vi "piezoUSBWriteWaveform.vi"(1 "positions (um)":dbl[](array[numeric])) -> ()   [LabVIEW 2017]
uses:
  globalDevices.vi
  Piezo/lvlib/Madlib.lvlib
panel:
  out "function return 2":i32
  out "Waveform Graph":dbl[](graph)
  out "function return":i32
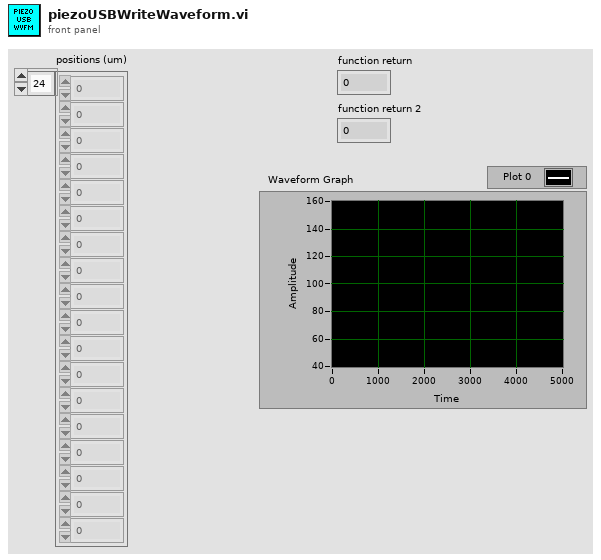
[diagram p1: front panel]
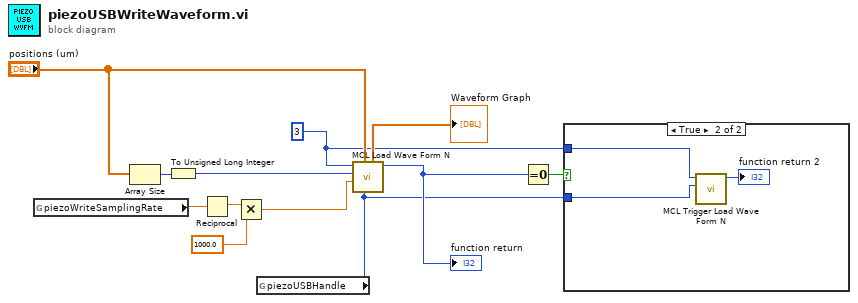
[diagram p0: block diagram]
diagram:
  w2 = u32 3 ("axis")
  n1 = global read "globalDevices.vi" "piezoWriteSamplingRate"() -> (w9:dbl)
  n2 = Array Size(array="positions (um)") -> (size(s)=w11:i32)
  n3 = To Unsigned Long Integer(number=w11) -> (unsigned 32bit integer=w10:u32)
  n4 = Reciprocal(x=w9) -> (1/x=w8:dbl)
  n5 = Multiply(x=w8, y=1000.0) -> (x*y=w6:dbl)
  n6 = global read "globalDevices.vi" "piezoUSBHandle"() -> (w1:i32)
  n7 = call "MCL Load Wave Form N.vi"("handle"=w1, "waveform"="positions (um)", "milliseconds"=w6, "DataPoints"=w10, "axis"=w2) -> ("function return"=w4:i32, "waveform out"=→"Waveform Graph":dbl[])  [unwired: 5 in]
  "function return" <- w4
  n8 = Equal To 0?(x=w4) -> (x = 0?=w3:bool)
  n9 = case shown="True" w3 {
    tunnel: w2 -> [_ w15]
    tunnel: w1 -> [_ w14]
    frame False {
    }
    frame True {
      n10 = call "MCL Trigger Load Wave Form N.vi"("handle"=w14, "axis"=w15) -> ("function return"=→"function return 2":i32)  [unwired: 9 in]
    }
  }
